vi "Read Module Top Layer.vi"(8 "error in (no error)":errorcluster, 11 "Module in":refnum<class "Module.lvclass">) -> (0 "error out":errorcluster, 2 "Module Top Layer":enum16{"Baseplate", "Kapton", "Sensor", "PCB"}(ring), 3 "Module out":refnum<class "Module.lvclass">)   [LabVIEW 2016, in "Module.lvclass"]
uses:
  Module.lvclass
  Module.lvclass/Module.ctl
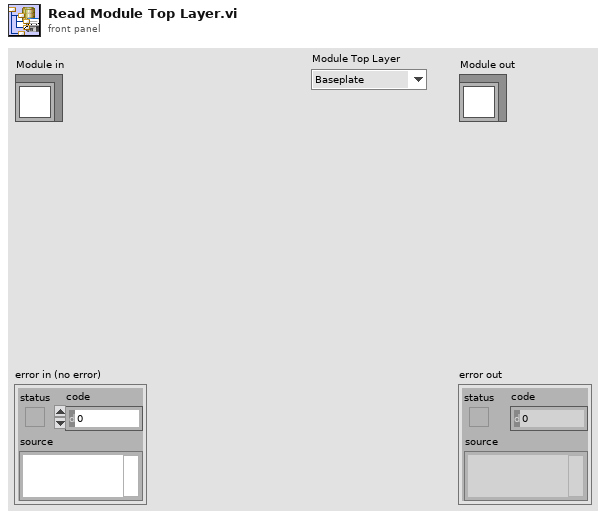
[diagram p1: front panel]
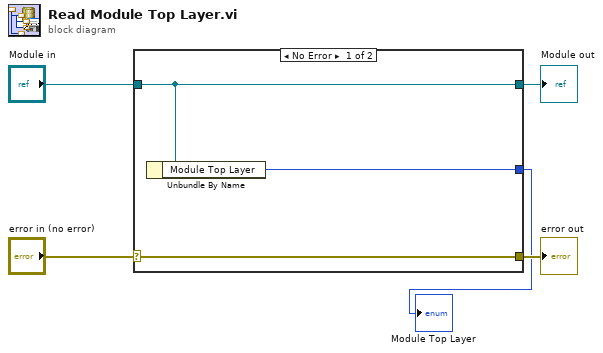
[diagram p0: block diagram]
diagram:
  n1 = case shown="No Error" "error in (no error)" {
    selector: "error in (no error)" -> [w8 w9]
    tunnel: [w8 w9] -> w4
    tunnel: [w7 w10] -> w2
    tunnel: "Module in" -> [w7 w10]
    tunnel: [w6 _] -> w1
    frame No Error {
      n2 = Unbundle By Name(w7) -> ("Module Top Layer"=w6:enum16{"Baseplate", "Kapton", "Sensor", "PCB"})
    }
    frame Error {
    }
  }
  "error out" <- w4
  "Module out" <- w2
  "Module Top Layer" <- w1
